vi "SetParam.vi"(8 "error in (no error)":errorcluster caption="entrée d'erreur (pas d'erreur)", 10 "pairwise_distances_argmin_min":T1={"axis"=1, "metric "="euclidean", "metric_kwargs"={"metric"=[], "kwargs"=[]}, "Returns"="argmin"}, 11 "Argmin_min.lvclass":refnum<class "Argmin_min.lvclass">) -> (0 "error out":errorcluster caption="sortie d'erreur", 3 "Argmin_min.lvclass":refnum<class "Argmin_min.lvclass">)   [LabVIEW 2020, in "Argmin_min.lvclass"]
doc: "Set Parameters"
uses:
  Argmin_min.lvclass
  Argmin_min.lvclass/Argmin_min.ctl
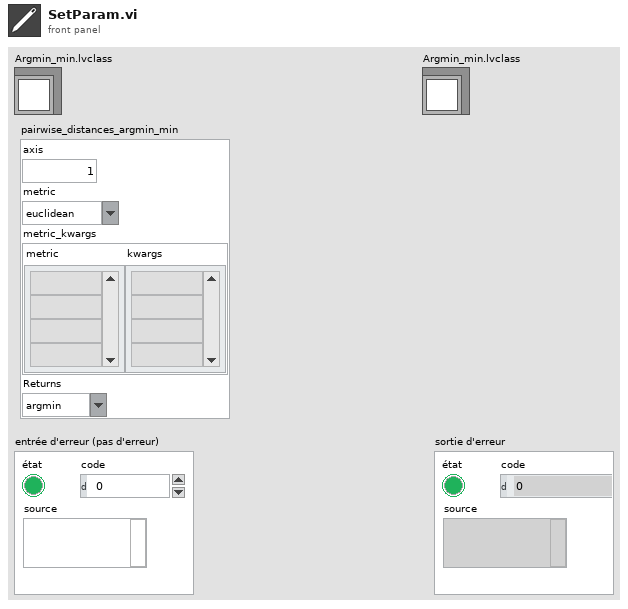
[diagram p1: front panel]
types:
  T1 = cluster{"axis":i32, "metric ":string, "metric_kwargs":cluster{"metric":string[], "kwargs":string[]}, "Returns":string}
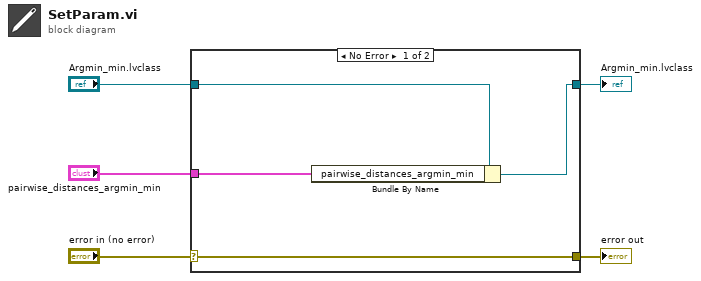
[diagram p0: block diagram]
diagram:
  n1 = case shown="No Error" "error in (no error)" {
    selector: "error in (no error)" -> [w9 w10]
    tunnel: [w9 w10] -> w4
    tunnel: [w7 w11] -> w2
    tunnel: "Argmin_min.lvclass" -> [w8 w11]
    tunnel: "pairwise_distances_argmin_min" -> [w6 _]
    frame No Error {
      n2 = Bundle By Name(cluster=w8, "pairwise_distances_argmin_min"=w6) -> (w7:refnum<class "Argmin_min.lvclass">)
    }
    frame Error {
    }
  }
  "error out" <- w4
  "Argmin_min.lvclass" <- w2
